vi "Sensor Test.vi"() -> ()   [LabVIEW 2011]
uses:
  <vilib>/DAQmx/read.llb/DAQmx Read (Analog DBL 1Chan 1Samp).vi
  <vilib>/DAQmx/create/channels.llb/DAQmx Create Channel (AI-Voltage-Basic).vi
  <vilib>/DAQmx/miscellaneous.llb/DAQmx Fill In Error Info.vi
panel:
  in  "physical channels":tag
  in  "stop":bool
  out "Voltage In":dbl(graph)
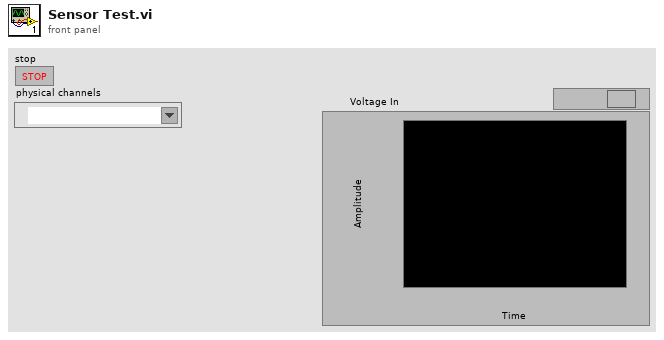
[diagram p1: front panel]
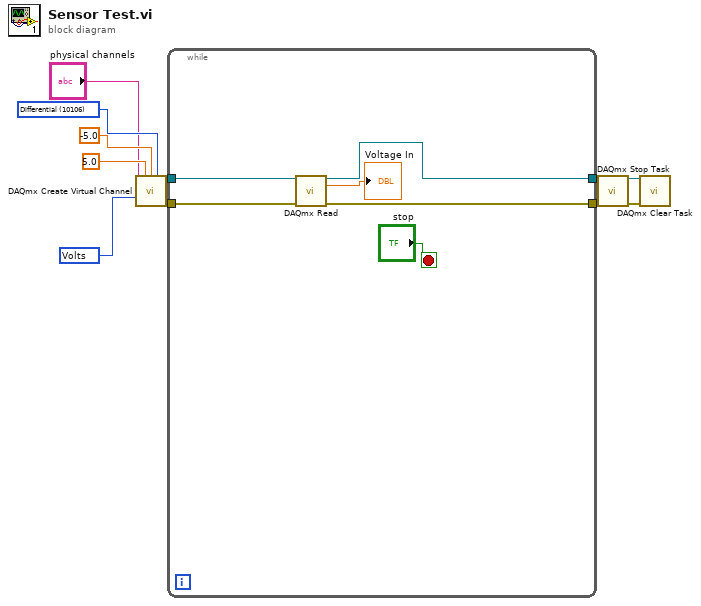
[diagram p0: block diagram]
diagram:
  w6 = 10106 items=["default"=-1, "RSE"=10083, "NRSE"=10078, "Differential"=10106, "Pseudodifferential"=12529] ("input terminal configuration")
  w11 = 10348 items=["Volts"=10348, "From Custom Scale"=10065] ("units")
  n1 = call-poly <vilib>:"DAQmx Create Virtual Channel.vi"("maximum value"=5.0, "minimum value"=-5.0, "input terminal configuration"=w6, "physical channels"="physical channels", "units"=w11) -> ("task out"=w7:refnum<k21>, "error out"=w8:errorcluster)  [unwired: 9 in]
  n2 = while {
    tunnel: w8 -> [w16]
    tunnel: w7 -> [w15]
    tunnel: [w14] -> w4
    tunnel: [w13] -> w5
    stop <- "stop" stop-if-true
    n3 = call-poly <vilib>:"DAQmx Read.vi"("task/channels in"=w15, "error in"=w16) -> ("task out"=w13:refnum<k21>, "data"=→"Voltage In":dbl, "error out"=w14:errorcluster)  [unwired: 11 in]
  }
  n4 = call <vilib>:"DAQmx Stop Task.vi"("task/channels in"=w5, "error in"=w4) -> ("task out"=w3:refnum<k21>, "error out"=w2:errorcluster)  [unwired: 12 in]
  n5 = call <vilib>:"DAQmx Clear Task.vi"("task in"=w3, "error in"=w2) -> ()  [unwired: 13 in, 1 out]
